vi "Numeric Output Item UI Update.vi"(8 "error in (no error)":errorcluster, 10 "Numeric UI Elements":T1, 11 "Output":T2) -> (0 "error out":errorcluster)   [LabVIEW 2015, in "OutputUI.lvclass"]
uses:
  OutputUI.lvclass
  Step/STEP_OUTPUT.ctl
  Step/OUTPUT_DATA_TYPE.ctl
  OUTPUT_CHECK_TYPE.ctl
  Step/OUTPUT_VALUE_TYPE.ctl
  Step.lvclass
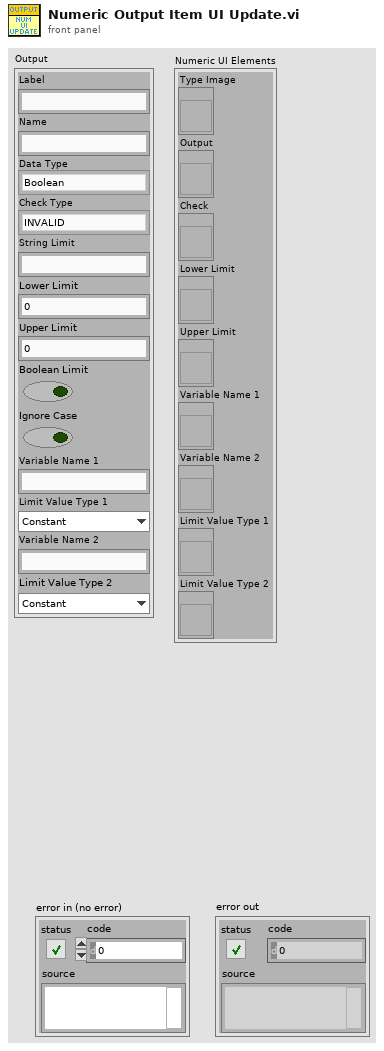
[diagram p1: front panel]
types:
  T1 = cluster{"Type Image":refnum<vi>, "Output":refnum<vi>, "Check":refnum<vi>, "Lower Limit":refnum<vi>, "Upper Limit":refnum<vi>, "Variable Name 1":refnum<vi>, "Variable Name 2":refnum<vi>, "Limit Value Type 1":refnum<vi>, "Limit Value Type 2":refnum<vi>}
  T2 = typedef "Step.lvclass/STEP_OUTPUT.ctl" = cluster{"Label":string, "Name":string, "Data Type":T3, "Check Type":T4, "String Limit":string, "Lower Limit":dbl, "Upper Limit":dbl, "Boolean Limit":bool, "Ignore Case":bool, "Variable Name 1":string, "Limit Value Type 1":T5, "Variable Name 2":string, "Limit Value Type 2":T5}
  T3 = typedef "Step.lvclass/OUTPUT_DATA_TYPE.ctl" = enum16{"Boolean", "String", "Numeric", "Other"}
  T4 = typedef "Step.lvclass/OUTPUT_CHECK_TYPE.ctl" = enum16{"INVALID", "DO_NOT_CHECK", "RECORD", "VARIABLE", "EQUAL", "NOT_EQUAL", "STR_CONTAINS", "STR_START_WITH", "STR_END_WITH", "STR_REGEX_MATCH", "NUM_GT", "NUM_LT", "NUM_GE", "NUM_LE", "NUM_RANGE", "NUM_RANGE_BDY"}
  T5 = typedef "Step.lvclass/OUTPUT_VALUE_TYPE.ctl" = enum16{"Constant", "Variable"}
  T6 = enum8{"Enabled", "Disabled", "Disabled and Grayed Out"}
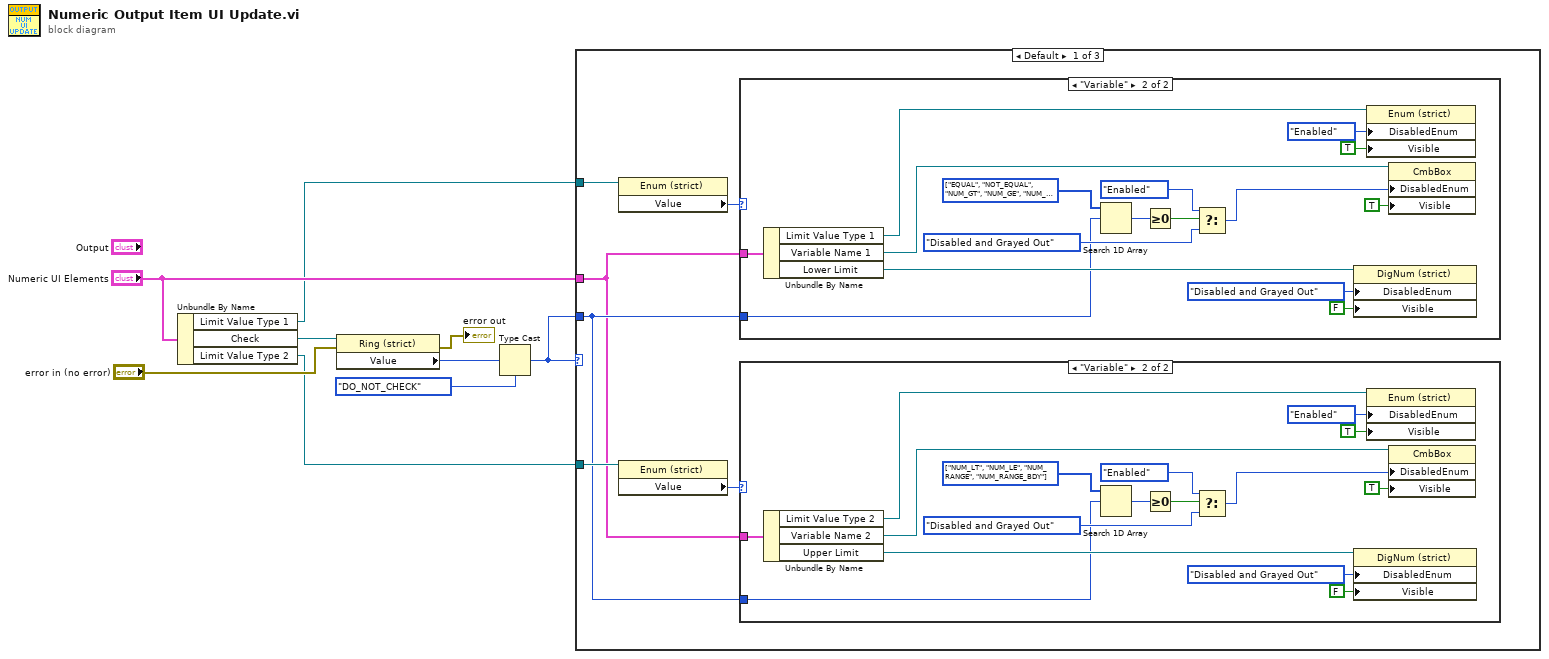
[diagram p0: block diagram]
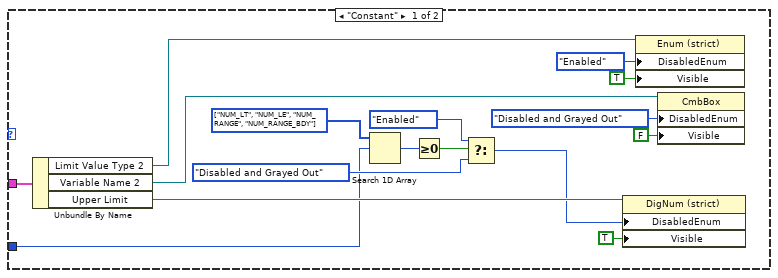
[diagram p2: hidden frame]
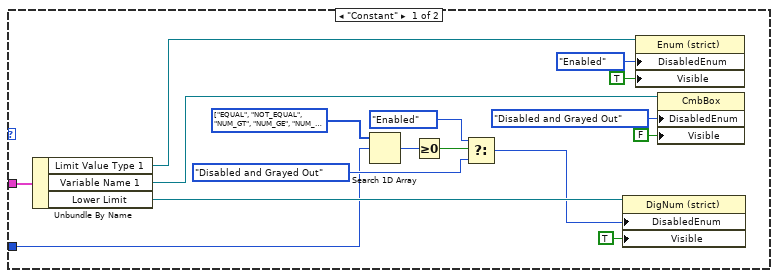
[diagram p3: hidden frame]
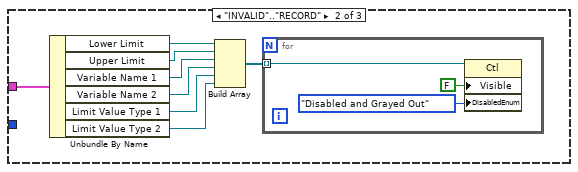
[diagram p4: hidden frame]
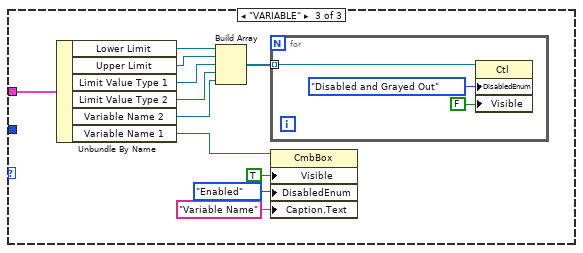
[diagram p5: hidden frame]
diagram:
  n1 = Unbundle By Name("Numeric UI Elements") -> ("Limit Value Type 1"=w3:refnum<vi>, "Check"=w9:refnum<vi>, "Limit Value Type 2"=w2:refnum<vi>)
  n2 = property class="Ring (strict)"(reference=w9, error in="error in (no error)") -> (error out=→"error out":errorcluster, "Value"=w7:u16)  [unwired: 1 out]
  n3 = Type Cast(type=OUTPUT_CHECK_TYPE."DO_NOT_CHECK" ("Check Type"), x=w7) -> (*(type *) &x=w4:T4)
  n4 = case shown="Default" w4 {
    tunnel: "Numeric UI Elements" -> [w10 w83 w101]
    tunnel: w4 -> [w11 _ _]
    tunnel: w3 -> [w14 _ _]
    tunnel: w2 -> [w12 _ _]
    frame Default {
      n5 = property class="Enum (strict)"(reference=w14) -> ("Value"=w15:T5)  [unwired: 1 in, 2 out]
      n6 = property class="Enum (strict)"(reference=w12) -> ("Value"=w13:T5)  [unwired: 1 in, 2 out]
      n7 = case shown="\"Variable\"" w15 {
        tunnel: w10 -> [w63 w79]
        tunnel: w11 -> [w56 w72]
        frame "Constant" {
          w61 = T4[] [enum."EQUAL", enum."NOT_EQUAL", enum."NUM_GT", enum."NUM_GE", enum."NUM_RANGE", enum."NUM_RANGE_BDY"] items=["INVALID", "DO_NOT_CHECK", "RECORD", "VARIABLE", "EQUAL", "NOT_EQUAL", "STR_CONTAINS", "STR_START_WITH", "STR_END_WITH", "STR_REGEX_MATCH", "NUM_GT", "NUM_LT", "NUM_GE", "NUM_LE", "NUM_RANGE", "NUM_RANGE_BDY"]
          n8 = Unbundle By Name(w63) -> ("Limit Value Type 1"=w48:refnum<vi>, "Variable Name 1"=w54:refnum<vi>, "Lower Limit"=w62:refnum<vi>)
          n9 = Search 1D Array(1D array=w61, element=w56) -> (index of element=w60:i32)  [unwired: 1 in]
          n10 = Greater Or Equal To 0?(x=w60) -> (x >= 0?=w59:bool)
          n11 = Select(t=T6."Enabled" ("f"), s=w59, f=T6."Disabled and Grayed Out") -> (s? t:f=w55:T6)
          n12 = property class="DigNum (strict)"(reference=w62, "DisabledEnum"=w55, "Visible"=TRUE) -> ()  [unwired: 1 in, 2 out]
          n13 = property class="Enum (strict)"(reference=w48, "DisabledEnum"=T6."Enabled" ("Disabled"), "Visible"=TRUE) -> ()  [unwired: 1 in, 2 out]
          n14 = property class="CmbBox"(reference=w54, "DisabledEnum"=T6."Disabled and Grayed Out" ("Disabled"), "Visible"=FALSE) -> ()  [unwired: 1 in, 2 out]
        }
        frame "Variable" {
          w77 = T4[] [enum."EQUAL", enum."NOT_EQUAL", enum."NUM_GT", enum."NUM_GE", enum."NUM_RANGE", enum."NUM_RANGE_BDY"] items=["INVALID", "DO_NOT_CHECK", "RECORD", "VARIABLE", "EQUAL", "NOT_EQUAL", "STR_CONTAINS", "STR_START_WITH", "STR_END_WITH", "STR_REGEX_MATCH", "NUM_GT", "NUM_LT", "NUM_GE", "NUM_LE", "NUM_RANGE", "NUM_RANGE_BDY"]
          n15 = Unbundle By Name(w79) -> ("Limit Value Type 1"=w66:refnum<vi>, "Variable Name 1"=w71:refnum<vi>, "Lower Limit"=w78:refnum<vi>)
          n16 = Search 1D Array(1D array=w77, element=w72) -> (index of element=w76:i32)  [unwired: 1 in]
          n17 = Greater Or Equal To 0?(x=w76) -> (x >= 0?=w75:bool)
          n18 = Select(t=T6."Enabled" ("f"), s=w75, f=T6."Disabled and Grayed Out") -> (s? t:f=w64:T6)
          n19 = property class="DigNum (strict)"(reference=w78, "DisabledEnum"=T6."Disabled and Grayed Out" ("f"), "Visible"=FALSE) -> ()  [unwired: 1 in, 2 out]
          n20 = property class="Enum (strict)"(reference=w66, "DisabledEnum"=T6."Enabled" ("Disabled"), "Visible"=TRUE) -> ()  [unwired: 1 in, 2 out]
          n21 = property class="CmbBox"(reference=w71, "DisabledEnum"=w64, "Visible"=TRUE) -> ()  [unwired: 1 in, 2 out]
        }
      }
      n22 = case shown="\"Variable\"" w13 {
        tunnel: w10 -> [w31 w47]
        tunnel: w11 -> [w24 w40]
        frame "Constant" {
          w29 = T4[] [enum."NUM_LT", enum."NUM_LE", enum."NUM_RANGE", enum."NUM_RANGE_BDY"] items=["INVALID", "DO_NOT_CHECK", "RECORD", "VARIABLE", "EQUAL", "NOT_EQUAL", "STR_CONTAINS", "STR_START_WITH", "STR_END_WITH", "STR_REGEX_MATCH", "NUM_GT", "NUM_LT", "NUM_GE", "NUM_LE", "NUM_RANGE", "NUM_RANGE_BDY"]
          n23 = Unbundle By Name(w31) -> ("Limit Value Type 2"=w16:refnum<vi>, "Variable Name 2"=w22:refnum<vi>, "Upper Limit"=w30:refnum<vi>)
          n24 = Search 1D Array(1D array=w29, element=w24) -> (index of element=w28:i32)  [unwired: 1 in]
          n25 = Greater Or Equal To 0?(x=w28) -> (x >= 0?=w27:bool)
          n26 = Select(t=T6."Enabled" ("f"), s=w27, f=T6."Disabled and Grayed Out") -> (s? t:f=w23:T6)
          n27 = property class="DigNum (strict)"(reference=w30, "DisabledEnum"=w23, "Visible"=TRUE) -> ()  [unwired: 1 in, 2 out]
          n28 = property class="Enum (strict)"(reference=w16, "DisabledEnum"=T6."Enabled" ("Disabled"), "Visible"=TRUE) -> ()  [unwired: 1 in, 2 out]
          n29 = property class="CmbBox"(reference=w22, "DisabledEnum"=T6."Disabled and Grayed Out" ("Disabled"), "Visible"=FALSE) -> ()  [unwired: 1 in, 2 out]
        }
        frame "Variable" {
          w45 = T4[] [enum."NUM_LT", enum."NUM_LE", enum."NUM_RANGE", enum."NUM_RANGE_BDY"] items=["INVALID", "DO_NOT_CHECK", "RECORD", "VARIABLE", "EQUAL", "NOT_EQUAL", "STR_CONTAINS", "STR_START_WITH", "STR_END_WITH", "STR_REGEX_MATCH", "NUM_GT", "NUM_LT", "NUM_GE", "NUM_LE", "NUM_RANGE", "NUM_RANGE_BDY"]
          n30 = Unbundle By Name(w47) -> ("Limit Value Type 2"=w34:refnum<vi>, "Variable Name 2"=w39:refnum<vi>, "Upper Limit"=w46:refnum<vi>)
          n31 = Search 1D Array(1D array=w45, element=w40) -> (index of element=w44:i32)  [unwired: 1 in]
          n32 = Greater Or Equal To 0?(x=w44) -> (x >= 0?=w43:bool)
          n33 = Select(t=T6."Enabled" ("f"), s=w43, f=T6."Disabled and Grayed Out") -> (s? t:f=w32:T6)
          n34 = property class="DigNum (strict)"(reference=w46, "DisabledEnum"=T6."Disabled and Grayed Out" ("f"), "Visible"=FALSE) -> ()  [unwired: 1 in, 2 out]
          n35 = property class="Enum (strict)"(reference=w34, "DisabledEnum"=T6."Enabled" ("Disabled"), "Visible"=TRUE) -> ()  [unwired: 1 in, 2 out]
          n36 = property class="CmbBox"(reference=w39, "DisabledEnum"=w32, "Visible"=TRUE) -> ()  [unwired: 1 in, 2 out]
        }
      }
    }
    frame "INVALID".."RECORD" {
      n37 = Unbundle By Name(w83) -> ("Lower Limit"=w87:refnum<vi>, "Upper Limit"=w86:refnum<vi>, "Variable Name 1"=w85:refnum<vi>, "Variable Name 2"=w82:refnum<vi>, "Limit Value Type 1"=w81:refnum<vi>, "Limit Value Type 2"=w80:refnum<vi>)
      n38 = Build Array(w87, w86, w85, w82, w81, w80) -> (w84:refnum<vi>[])
      n39 = for {
        tunnel: w84 -> [w90] mode=indexing
        n40 = property class="Ctl"(reference=w90, "Visible"=FALSE, "DisabledEnum"=T6."Disabled and Grayed Out" ("Disabled")) -> ()  [unwired: 1 in, 2 out]
      }
    }
    frame "VARIABLE" {
      n41 = Unbundle By Name(w101) -> ("Lower Limit"=w100:refnum<vi>, "Upper Limit"=w99:refnum<vi>, "Limit Value Type 1"=w94:refnum<vi>, "Limit Value Type 2"=w93:refnum<vi>, "Variable Name 2"=w92:refnum<vi>, "Variable Name 1"=w91:refnum<vi>)
      n42 = Build Array(w100, w99, w94, w93, w92) -> (w98:refnum<vi>[])
      n43 = for {
        tunnel: w98 -> [w104] mode=indexing
        n44 = property class="Ctl"(reference=w104, "DisabledEnum"=T6."Disabled and Grayed Out" ("Disabled"), "Visible"=FALSE) -> ()  [unwired: 1 in, 2 out]
      }
      n45 = property class="CmbBox"(reference=w91, "Visible"=TRUE, "DisabledEnum"=T6."Enabled" ("Disabled"), "Caption.Text"="Variable Name" ("format string")) -> ()  [unwired: 1 in, 2 out]
    }
  }
